vi "Channel Simu.vi"(6 "Error Feedback":bool[](array[boolean]), 7 "Temperature Feedback":dbl[](array[numeric]) format="%#_13g", 8 "Flow Feedback":dbl[](array[numeric]) format="%#_13g", 9 "Pressure Feedback":dbl[](array[numeric]) format="%#_13g", 10 "Channels":T2(array[cluster]), 11 "Iteration Interval (s)":dbl) -> (0 "Flow Feedback Out":dbl[](array[numeric]), 1 "Pressure Feedback Out":dbl[](array[numeric]), 2 "Temperature Feedback Out":dbl[](array[numeric]), 3 "Channels Out":T1[](array[typedef]), 4 "Error Feedback Out":bool[](array[boolean]))   [LabVIEW 2023]
uses:
  C:/Program Files/National Instruments/AMS plugin/Capabilities/Capabilities/High Level Capabilities/Chiller Cluster/Producer Ch.ctl
  C:/Program Files/National Instruments/AMS plugin/Capabilities/Capabilities/High Level Capabilities/Chiller Cluster/Chiller Cluster.lvclass
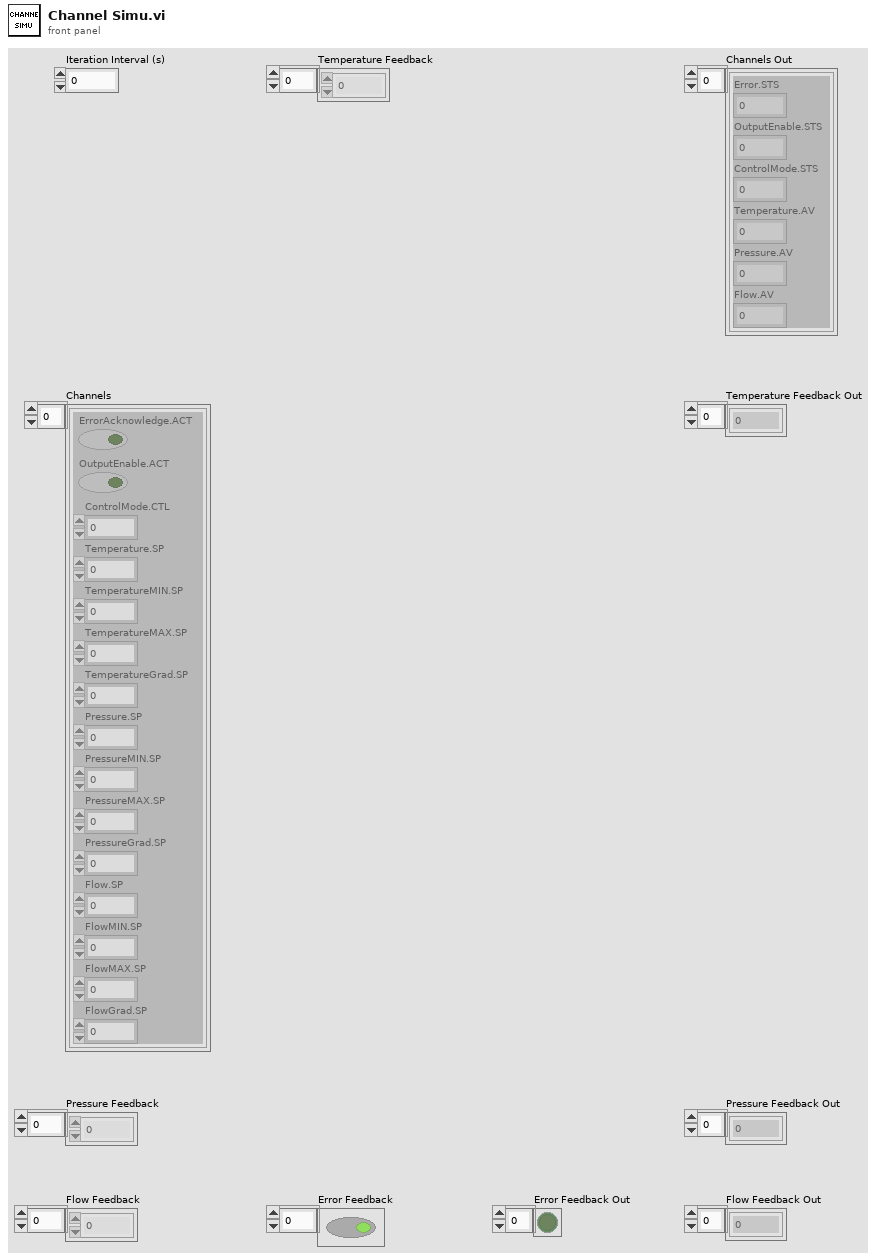
[diagram p1: front panel]
types:
  T1 = typedef "Chiller Cluster.lvclass/Producer Ch.ctl" = cluster{"Error.STS":i32, "OutputEnable.STS":i32, "ControlMode.STS":u16, "Temperature.AV":dbl, "Pressure.AV":dbl, "Flow.AV":dbl}
  T2 = cluster{"ErrorAcknowledge.ACT":bool, "OutputEnable.ACT":bool, "ControlMode.CTL":u16, "Temperature.SP":dbl, "TemperatureMIN.SP":dbl, "TemperatureMAX.SP":dbl, "TemperatureGrad.SP":dbl, "Pressure.SP":dbl, "PressureMIN.SP":dbl, "PressureMAX.SP":dbl, "PressureGrad.SP":dbl, "Flow.SP":dbl, "FlowMIN.SP":dbl, "FlowMAX.SP":dbl, "FlowGrad.SP":dbl}[]
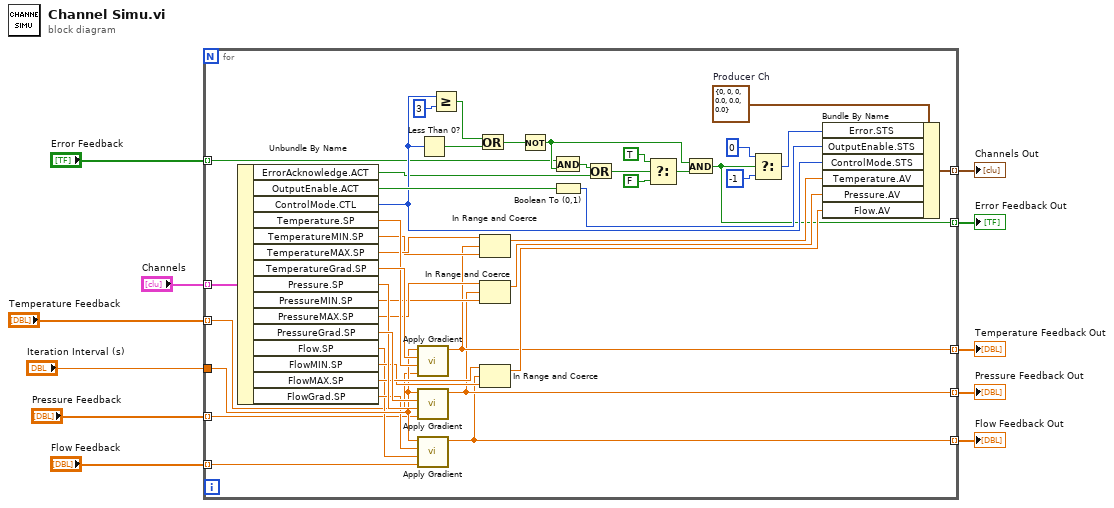
[diagram p0: block diagram]
diagram:
  n1 = for {
    tunnel: "Channels" -> [w55] mode=indexing
    tunnel: "Iteration Interval (s)" -> [w44]
    tunnel: [w21] -> w4 mode=indexing
    tunnel: "Temperature Feedback" -> [w19] mode=indexing
    tunnel: "Pressure Feedback" -> [w18] mode=indexing
    tunnel: "Flow Feedback" -> [w17] mode=indexing
    tunnel: "Error Feedback" -> [w16] mode=indexing
    tunnel: [w12] -> w5 mode=indexing
    tunnel: [w15] -> w3 mode=indexing
    tunnel: [w14] -> w2 mode=indexing
    tunnel: [w13] -> w1 mode=indexing
    w40 = T1 {"Error.STS"=0, "OutputEnable.STS"=0, "ControlMode.STS"=0, "Temperature.AV"=0.0, "Pressure.AV"=0.0, "Flow.AV"=0.0}  # Producer Ch
    n2 = Unbundle By Name(w55) -> ("ErrorAcknowledge.ACT"=w24:bool, "OutputEnable.ACT"=w41:bool, "ControlMode.CTL"=w32:u16, "Temperature.SP"=w53:dbl, "TemperatureMIN.SP"=w51:dbl, "TemperatureMAX.SP"=w52:dbl, "TemperatureGrad.SP"=w54:dbl, "Pressure.SP"=w49:dbl, "PressureMIN.SP"=w47:dbl, "PressureMAX.SP"=w48:dbl, "PressureGrad.SP"=w50:dbl, "Flow.SP"=w42:dbl, "FlowMIN.SP"=w45:dbl, "FlowMAX.SP"=w46:dbl, "FlowGrad.SP"=w43:dbl)
    n3 = call "Apply Gradient.vi"("Reminder"=w19, "Setpoint"=w53, "Gradient"=w54, "Iteration Interval"=w44) -> ("Current Setpoint"=w15:dbl)  [unwired: 7 in]
    n4 = call "Apply Gradient.vi"("Reminder"=w18, "Setpoint"=w49, "Gradient"=w50, "Iteration Interval"=w44) -> ("Current Setpoint"=w14:dbl)  [unwired: 7 in]
    n5 = call "Apply Gradient.vi"("Reminder"=w17, "Setpoint"=w42, "Gradient"=w43, "Iteration Interval"=w44) -> ("Current Setpoint"=w13:dbl)  [unwired: 7 in]
    n6 = Less Than 0?(x=w32) -> (x < 0?=w34:bool)
    n7 = Greater Or Equal?(x=w32, y=u16 3) -> (x >= y?=w35:bool)
    n8 = Or(x=w35, y=w34) -> (x .or. y?=w20:bool)
    n9 = In Range and Coerce(upper limit=w52, x=w15, lower limit=w51) -> (coerced(x)=w38:dbl)  [unwired: 1 out]
    n10 = In Range and Coerce(upper limit=w48, x=w14, lower limit=w47) -> (coerced(x)=w37:dbl)  [unwired: 1 out]
    n11 = In Range and Coerce(upper limit=w46, x=w13, lower limit=w45) -> (coerced(x)=w36:dbl)  [unwired: 1 out]
    n12 = Not(x=w20) -> (.not. x?=w23:bool)
    n13 = And(x=w16, y=w23) -> (x .and. y?=w25:bool)
    n14 = Boolean To (0,1)(Boolean=w41) -> (0, 1=w39:i16)
    n15 = Or(x=w25, y=w24) -> (x .or. y?=w29:bool)
    n16 = Select(t=TRUE, s=w29, f=FALSE) -> (s? t:f=w26:bool)
    n17 = And(x=w23, y=w26) -> (x .and. y?=w12:bool)
    n18 = Select(t=0, s=w12, f=-1) -> (s? t:f=w22:i32)
    n19 = Bundle By Name(cluster=w40, "Error.STS"=w22, "OutputEnable.STS"=w39, "ControlMode.STS"=w32, "Temperature.AV"=w38, "Pressure.AV"=w37, "Flow.AV"=w36) -> (w21:T1)
  }
  "Error Feedback Out" <- w5
  "Channels Out" <- w4
  "Temperature Feedback Out" <- w3
  "Pressure Feedback Out" <- w2
  "Flow Feedback Out" <- w1
